vi "DeadZone.vi"(10 "Turn":dbl, 11 "Speed":dbl) -> (2 "Turn  Out":dbl, 3 "Speed Out":dbl)   [LabVIEW 2014]
panel:
  in  "Turn Deadzone":dbl=0.05
  in  "Speed Deadzone":dbl=0.2
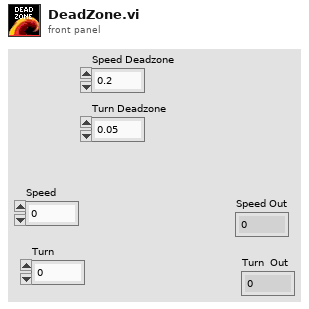
[diagram p1: front panel]
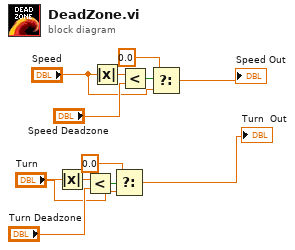
[diagram p0: block diagram]
diagram:
  n1 = Absolute Value(x="Turn") -> (abs(x)=w10:dbl)
  n2 = Less?(x=w10, y="Turn Deadzone") -> (x < y?=w7:bool)
  n3 = Absolute Value(x="Speed") -> (abs(x)=w12:dbl)
  n4 = Select(t=0.0, s=w7, f="Turn") -> (s? t:f=→"Turn  Out":dbl)
  n5 = Less?(x=w12, y="Speed Deadzone") -> (x < y?=w8:bool)
  n6 = Select(t=0.0, s=w8, f="Speed") -> (s? t:f=→"Speed Out":dbl)
